vi "Test File Sink Default Logger.vi"(11 "Test Case In":refnum<class "File Sink.lvclass">) -> (0 "error out":errorcluster, 3 "Test Case Out":refnum<class "File Sink.lvclass">)   [LabVIEW 2020, in "Testing.lvlib" / "File Sink.lvclass"]
uses:
  File Sink.lvclass
  C:/Program Files (x86)/National Instruments/LabVIEW 2020/vi.lib/Astemes/LUnit/Test Case.lvclass
  Source/Type Defs/Debug Level.ctl
  <vilib>/Astemes/LUnit/Test Case.lvclass/Test Case.ctl
  e94ff1bf-c1b1-42c1-a6e3-1538fdc900a3.vi
  4993e8ee-a06a-463a-9684-69129f64d5ce.vi
  ebeb964f-1c40-45c4-b7ad-328f89dac856.vi
  <vilib>/Astemes/LUnit/Core/LUnit Test Case/Private/Append Pass Result.vi
  <vilib>/Astemes/LUnit/Core/LUnit Test Case/Private/Append Fail Result.vi
  e94ff1bf-c1b1-42c1-a6e3-1538fdc900a3.vi/9c5d11cd-9439-4240-a1ee-d9baace9c924.vi
  4993e8ee-a06a-463a-9684-69129f64d5ce.vi/9c5d11cd-9439-4240-a1ee-d9baace9c924.vi
  ebeb964f-1c40-45c4-b7ad-328f89dac856.vi/9c5d11cd-9439-4240-a1ee-d9baace9c924.vi
  <vilib>/Astemes/LUnit/Core/LUnit Test Case/Private/Run In UI.vi
  <vilib>/Utility/error.llb/Clear Errors.vi
  Source/Sinks/File Sink/File Sink.lvclass
  C:/Users/hughe_cx/Documents/05_repos/LVLog/Source/Sinks/Sink/Sink.lvclass
  <vilib>/Astemes/LUnit/Test Case.lvclass
  Source/LV Log.lvlib
  Source/Logger/Logger.lvclass
  Testing.lvlib
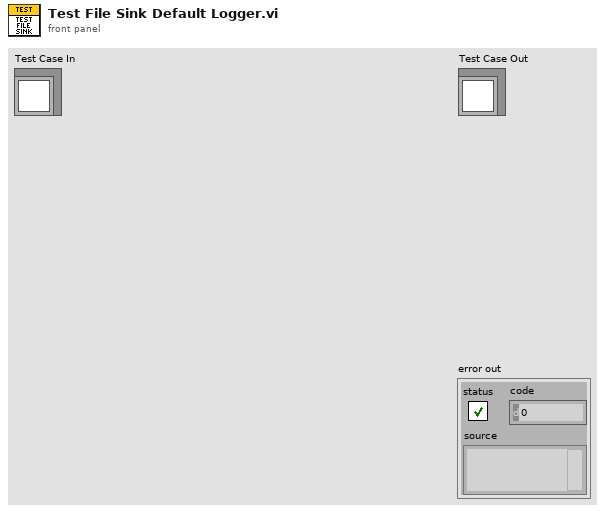
[diagram p1: front panel]
types:
  T1 = typedef "LV Log.lvlib/Debug Level.ctl" = enum16{"DEFAULT", "DEBUG", "INFO", "WARN", "ERROR", "FATAL"}
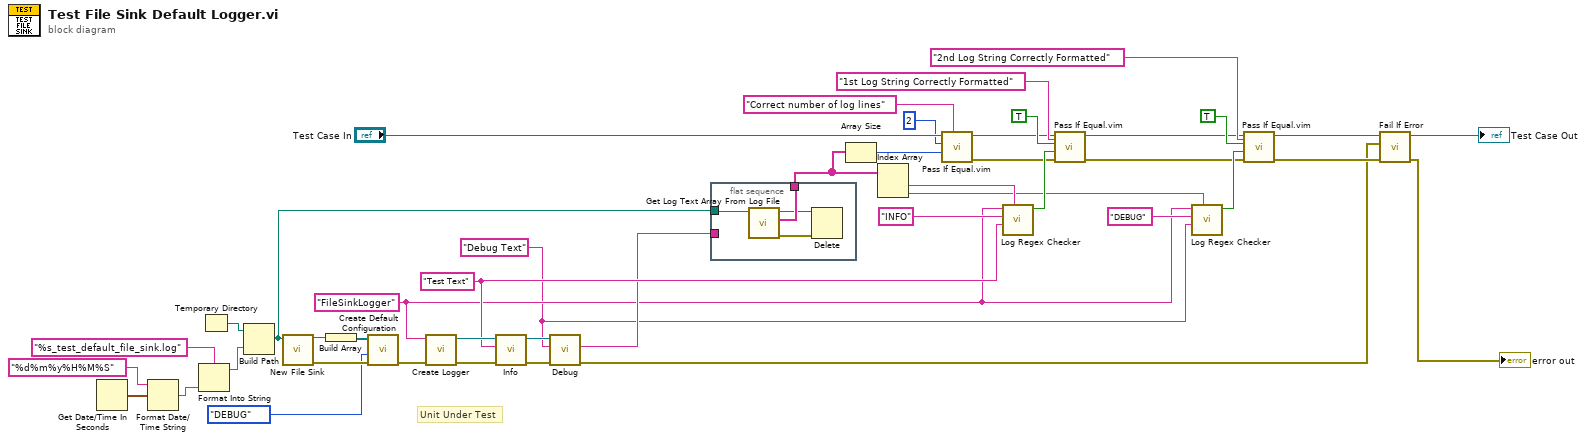
[diagram p0: block diagram]
diagram:
  w16 = "Debug Text" ("Log Text")
  w27 = "Test Text" ("Log Text")
  w17 = "FileSinkLogger" ("Name")
  # "Unit Under Test"
  n1 = Get Date/Time In Seconds() -> (seconds since 1Jan1904=w36:timestamp)
  n2 = Format Date/Time String(time format string (%c)="%d%m%y%H%M%S", seconds (now)=w36) -> (date/time string=w34:string)  [unwired: 1 in]
  n3 = Format Into String(format string="%s_test_default_file_sink.log", w34) -> (resulting string=w37:string)  [unwired: 2 in, 1 out]
  n4 = Temporary Directory() -> (w39:path)
  n5 = Build Path(base path=w39, name or relative path=w37) -> (appended path=w30:path)
  n6 = call "New File Sink.vi"("File Path"=w30) -> ("error out"=w41:errorcluster, "File Sink out"=w1:refnum<class "File Sink.lvclass">)  [unwired: 9 in]
  n7 = Build Array(w1) -> (w40:refnum<class "File Sink.lvclass">[])
  n8 = call "Create Default Configuration.vi"("Sinks"=w40, "Debug Level in"=Debug_Level."DEBUG", "error in (no error)"=w41) -> ("error out"=w42:errorcluster)  [unwired: 7 in]
  n9 = call "Create Logger.vi"("error in (no error)"=w42, "Name"=w17) -> ("error out"=w32:errorcluster, "Logger out"=w31:refnum<class "Logger.lvclass">)  [unwired: 8 in]
  n10 = call "Info.vi"("error in (no error)"=w32, "Log Text"=w27, "Logger in"=w31) -> ("error out"=w26:errorcluster, "Logger out"=w25:refnum<class "Logger.lvclass">)  [unwired: 6 in, 1 out]
  n11 = call "Debug.vi"("error in (no error)"=w26, "Log Text"=w16, "Logger in"=w25) -> ("error out"=w2:errorcluster, "Log Output"=w24:string)  [unwired: 6 in, 1 out]
  n12 = flat-sequence {
    tunnel: w30 -> [w48]
    tunnel: w24 -> [_]
    tunnel: [w47] -> w9
    frame #0 {
      n13 = call "Get Log Text Array From Log File.vi"("Log File Path in"=w48) -> ("error out"=w46:errorcluster, "Log Text Array"=w47:string[], "Log File Path out"=w45:path)  [unwired: 8 in]
      n14 = Delete(path (use dialog)=w45, error in=w46) -> ()  [unwired: 3 in, 3 out]
    }
  }
  n15 = Array Size(array=w9) -> (size(s)=w8:i32)
  n16 = Index Array(array=w9) -> (element #1=w15:string, element #2=w14:string)  [unwired: 2 in]
  n17 = call "Pass If Equal.vim"("Description"="Correct number of log lines", "Actual"=w8, "Expected"=2, "LUnit Test Case In"="Test Case In") -> ("error out"=w3:errorcluster, "LUnit Test Case Out"=w11:refnum<class "File Sink.lvclass">)  [unwired: 6 in]
  n18 = call "Log Regex Checker.vi"("Log String"=w15, "Expected Log Text (Any)"=w27, "Expected Log Level (Any)"="INFO", "Expected Logger Name (Any)"=w17) -> ("Math Found"=w22:bool)  [unwired: 5 in, 2 out]
  n19 = call "Pass If Equal.vim"("Description"="1st Log String Correctly Formatted", "error in (no error)"=w3, "Actual"=w22, "Expected"=TRUE, "LUnit Test Case In"=w11) -> ("error out"=w4:errorcluster, "LUnit Test Case Out"=w13:refnum<class "File Sink.lvclass">)  [unwired: 5 in]
  n20 = call "Log Regex Checker.vi"("Log String"=w14, "Expected Log Text (Any)"=w16, "Expected Log Level (Any)"="DEBUG", "Expected Logger Name (Any)"=w17) -> ("Math Found"=w21:bool)  [unwired: 5 in, 2 out]
  n21 = call "Pass If Equal.vim"("Description"="2nd Log String Correctly Formatted", "error in (no error)"=w4, "Actual"=w21, "Expected"=TRUE, "LUnit Test Case In"=w13) -> ("error out"=w5:errorcluster, "LUnit Test Case Out"=w12:refnum<class "File Sink.lvclass">)  [unwired: 5 in]
  n22 = call <vilib>:"Fail If Error.vi"("error in (no error)"=w5, "Assert error"=w2, "LUnit Test Case In"=w12) -> ("error out"=→"error out":errorcluster, "LUnit Test Case Out"=→"Test Case Out":refnum<class "File Sink.lvclass">)  [unwired: 7 in]
